vi "Remove Trailing Zeros.vi"(1 "String In":string) -> (0 "String Out":string)   [LabVIEW 2013]
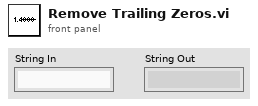
[diagram p1: front panel]
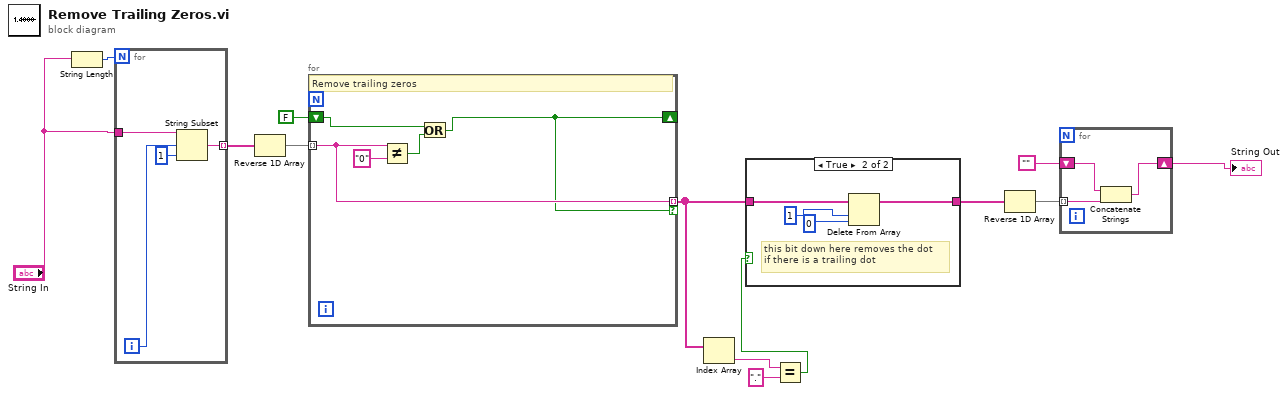
[diagram p0: block diagram]
diagram:
  n1 = String Length(string="String In") -> (length=w6:i32)
  n2 = for {
    N: w6 -> [_]
    tunnel: "String In" -> [w17]
    tunnel: [w14] -> w8 mode=indexing
    i -> [w16]
    n3 = String Subset(string=w17, offset (0)=w16, length (rest)=1 ("length (rest)")) -> (substring=w14:string)
  }
  n4 = Reverse 1D Array(array=w8) -> (reversed array=w9:string[])
  n5 = for {
    tunnel: w9 -> [w19] mode=indexing
    shift-right: [w18] -> _
    shift-left: FALSE -> [w20]
    tunnel: [w19] -> w2 mode=indexing if=w18
    # "Remove trailing zeros"
    n6 = Not Equal?(x=w19, y="0") -> (x != y?=w21:bool)
    n7 = Or(x=w20, y=w21) -> (x .or. y?=w18:bool)
  }
  n8 = Index Array(array=w2) -> (element=w5:string)  [unwired: 1 in]
  n9 = Equal?(x=w5, y=".") -> (x = y?=w3:bool)
  n10 = case shown="True" w3 {
    tunnel: w2 -> [w23 w27]
    tunnel: [w23 w26] -> w1
    frame False {
    }
    frame True {
      # "this bit down here removes the dot\nif there is a trailing dot"
      n11 = Delete From Array(array=w27, length=1, index=0) -> (array with subset deleted=w26:string[])  [unwired: 1 out]
    }
  }
  n12 = Reverse 1D Array(array=w1) -> (reversed array=w11:string[])
  n13 = for {
    tunnel: w11 -> [w30] mode=indexing
    shift-right: [w28] -> w13
    shift-left: "" -> [w29]
    n14 = Concatenate Strings(w29, w30) -> (w28:string)
  }
  "String Out" <- w13
